vi "SCMP CoMP-S Mechanism - rotation2.vi"(8 "error in (no error)":errorcluster, 9 "Auto Motors":bool, 10 "Old Rotation":dbl, 11 "Desired Rotation":dbl) -> (0 "error out":errorcluster, 3 "Rotation out":dbl)   [LabVIEW 2014]
panel:
  # "Moving Rotation\n     wait please"
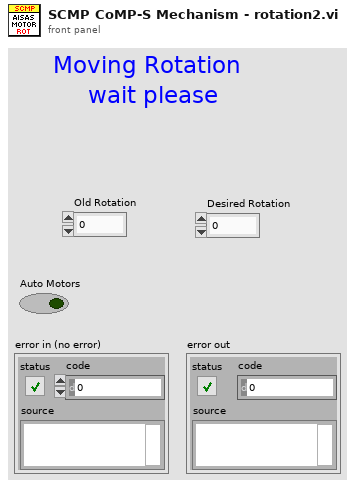
[diagram p1: front panel]
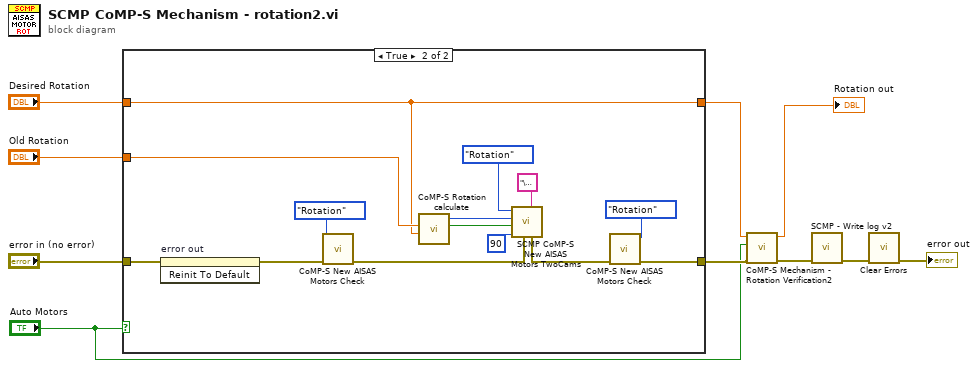
[diagram p0: block diagram]
diagram:
  n1 = case shown="True" "Auto Motors" {
    tunnel: "error in (no error)" -> [w12 w26]
    tunnel: "Old Rotation" -> [_ w18]
    tunnel: [w12 w19] -> w4
    tunnel: "Desired Rotation" -> [w11 w17]
    tunnel: [w11 w17] -> w3
    frame False {
    }
    frame True {
      n2 = invoke on="error out" class="Clust (strict)" method="Reinit To Default"(error in=w26) -> (error out=w20:errorcluster)  [unwired: 2 in, 2 out]
      n3 = call "CoMP-S New AISAS Motors Check.vi"("error in (no error)"=w20, "Motor selection"=enum32{"Rotation", "Difuser ", "Objective Lens"}."Rotation") -> ("error out"=w15:errorcluster)  [unwired: 9 in]
      n4 = call "CoMP-S Rotation calculate.vi"("New Value"=w17, "Old Value"=w18) -> ("Direction"=w13:bool, "steps"=w14:i32)  [unwired: 6 in, 2 out]
      n5 = call "SCMP CoMP-S New AISAS Motors TwoCams.vi"("Motion Code"="\u0002", "error in (no error)"=w15, "steps/sec"=u32 90, "motor rotation"=w13, "Steps"=w14, "Motor selection"=enum32{"Rotation", "Difuser ", "Objective Lens"}."Rotation") -> ("error out"=w23:errorcluster)  [unwired: 2 in, 3 out]
      n6 = call "CoMP-S New AISAS Motors Check.vi"("error in (no error)"=w23, "Motor selection"=enum32{"Rotation", "Difuser ", "Objective Lens"}."Rotation") -> ("error out"=w19:errorcluster)  [unwired: 9 in]
    }
  }
  n7 = call "CoMP-S Mechanism - Rotation Verification2.vi"("error in (no error)"=w4, "Motors"="Auto Motors", "Rotation"=w3) -> ("error out"=w5:errorcluster, "Rotation out"=→"Rotation out":dbl)  [unwired: 7 in]
  n8 = call "SCMP - Write log v2.vi"("Error to log"=w5) -> ("error out"=w8:errorcluster)  [unwired: 8 in, 2 out]
  n9 = call <vilib>:"Clear Errors.vi"("error in (no error)"=w8) -> ("error out"=→"error out":errorcluster)  [unwired: 5 in, 1 out]
